vi "Move Stage 2.vi"() -> ()   [LabVIEW 2016]
uses:
  C:/Program Files/Newport/Piezo Motion Control/Newport AG-UC2-UC8 Applet/Bin/AgilisCmdLib.DLL
  Program Files/Newport/Piezo Motion Control/Newport AG-UC2-UC8 Applet/Bin/AgilisCmdLib.DLL
panel:
  out "errstring 3":string
  in  "stop":bool
  in  "Boolean":bool
  in  "Step Speed":i64
  in  "Stage Address":i32
  out "errstring":string
  out "error out":errorcluster={"status"=TRUE, "code"=1172, "source"="Invoke Node Error calling method Newport.AgilisCmdLib.AgilisCmds.ML, (System.ArgumentNullException: Key cannot be null.\r\nParameter name: key) <append><b>System.ArgumentNullException</b> in move_stage.vi"}
  out "ControllerVersion":string="AG-UC2 v2.2.0"
  out "VE":i32
  in  "Instrument Key":string="COM9"
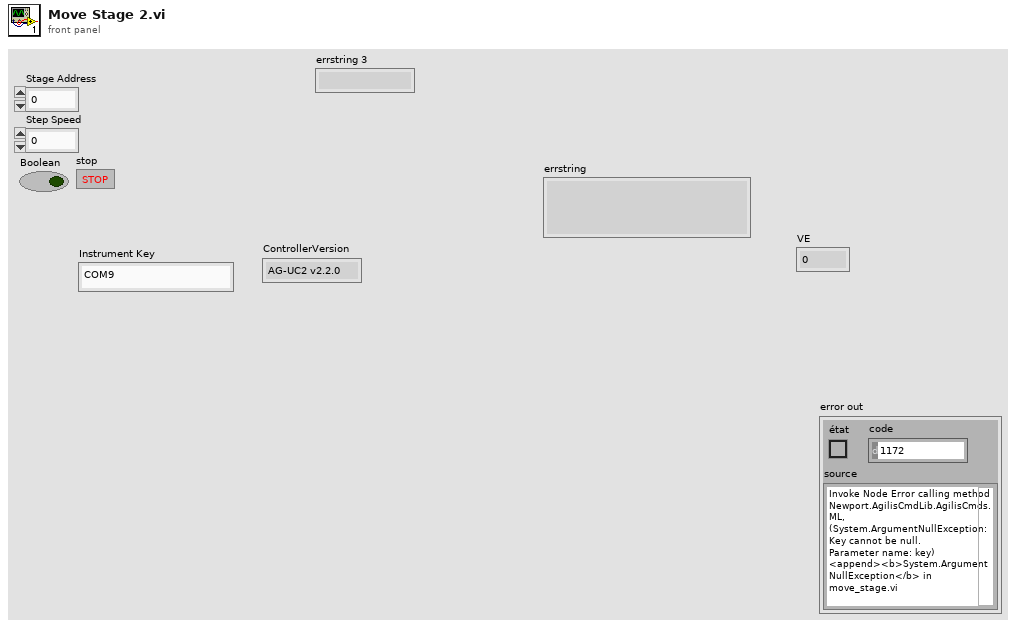
[diagram p1: front panel]
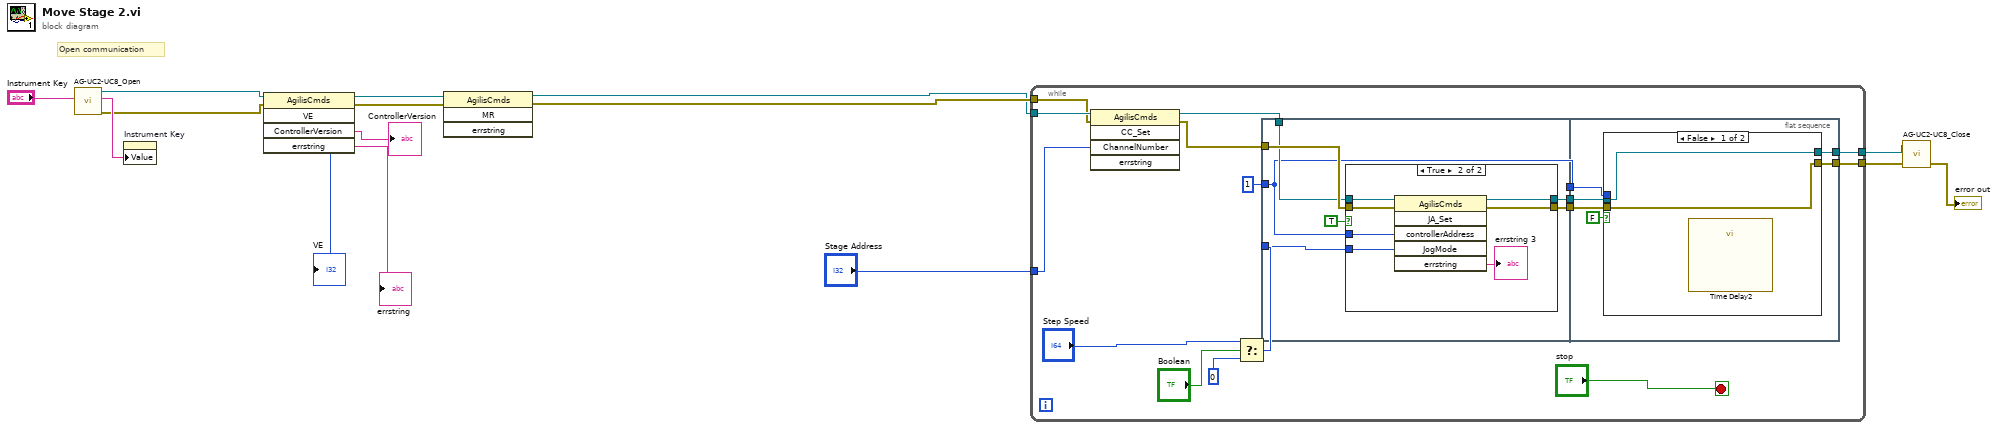
[diagram p0: block diagram]
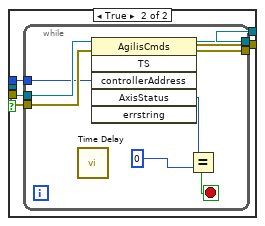
[diagram p3: hidden frame]
diagram:
  # "Open communication"
  n1 = call "AG-UC2-UC8_Open.vi"("Instrument Key IN"="Instrument Key") -> ("error out"=w13:errorcluster, "Instrument Key OUT"=w14:string, "AG-UC2-UC8 Reference"=w12:refnum<k24>)  [unwired: 3 in, 1 out]
  n2 = property on="Instrument Key" class="Str"("Value"=w14) -> ()  [unwired: 2 in, 2 out]
  n3 = invoke class="AgilisCmds" method="VE"(reference=w12, error in=w13) -> (reference out=w9:refnum<k24>, error out=w8:errorcluster, "VE"=→"VE":i32, "ControllerVersion"=→"ControllerVersion":string, "errstring"=→"errstring":string)  [unwired: 3 in]
  n4 = invoke class="AgilisCmds" method="MR"(reference=w9, error in=w8) -> (reference out=w2:refnum<k24>, error out=w3:errorcluster)  [unwired: 2 in, 2 out]
  n5 = while {
    tunnel: [w28] -> w5
    tunnel: [w27] -> w4
    tunnel: w2 -> [w22]
    tunnel: w3 -> [w21]
    tunnel: "Stage Address" -> [w17]
    stop <- "stop" stop-if-true
    n6 = invoke class="AgilisCmds" method="CC_Set"(reference=w22, error in=w21, "ChannelNumber"=w17) -> (reference out=w20:refnum<k24>, error out=w19:errorcluster)  [unwired: 2 in, 3 out]
    n7 = Select(t="Step Speed", s="Boolean", f=i64 0) -> (s? t:f=w23:i64)
    n8 = flat-sequence {
      tunnel: w19 -> [w38]
      tunnel: w20 -> [w37]
      tunnel: 1 ("controllerAddress") -> [w33]
      tunnel: w23 -> [w36]
      tunnel: [w35] -> w31
      tunnel: [w34] -> w30
      tunnel: [w33] -> w26
      tunnel: w31 -> [w53]
      tunnel: w30 -> [w52]
      tunnel: [w51] -> w28
      tunnel: [w50] -> w27
      tunnel: w26 -> [w49]
      frame #0 {
        n9 = case shown="True" TRUE {
          tunnel: w38 -> [w39 w47]
          tunnel: w37 -> [w40 w46]
          tunnel: w33 -> [_ w45]
          tunnel: w36 -> [_ w41]
          tunnel: [w40 w44] -> w35
          tunnel: [w39 w43] -> w34
          frame False {
          }
          frame True {
            n10 = invoke class="AgilisCmds" method="JA_Set"(reference=w46, error in=w47, "controllerAddress"=w45, "JogMode"=w41) -> (reference out=w44:refnum<k24>, error out=w43:errorcluster, "errstring"=→"errstring 3":string)  [unwired: 2 in, 3 out]
          }
        }
      }
      frame #1 {
        n11 = case shown="False" FALSE {
          tunnel: w53 -> [w55 w60]
          tunnel: w52 -> [w54 w59]
          tunnel: [w54 w58] -> w51
          tunnel: [w55 w57] -> w50
          tunnel: w49 -> [_ w56]
          frame False {
            n12 = call "Time Delay2"() -> ()  [unwired: 11 in, 1 out]
          }
          frame True {
            n13 = while {
              tunnel: w60 -> [w65]
              tunnel: w59 -> [w64]
              tunnel: [w63] -> w58
              tunnel: [w62] -> w57
              tunnel: w56 -> [w61]
              stop <- w68 stop-if-true
              n14 = call "Time Delay"() -> ()  [unwired: 11 in, 1 out]
              n15 = invoke class="AgilisCmds" method="TS"(reference=w65, error in=w64, "controllerAddress"=w61) -> (reference out=w62:refnum<k24>, error out=w63:errorcluster, "AxisStatus"=w67:i32)  [unwired: 3 in, 3 out]
              n16 = Equal?(x=w67, y=0) -> (x = y?=w68:bool)
            }
          }
        }
      }
    }
  }
  n17 = call "AG-UC2-UC8_Close.vi"("error in (no error)"=w5, "AG-UC2-UC8 Reference"=w4) -> ("Error out"=→"error out":errorcluster)  [unwired: 2 in, 1 out]
